vi "PH_ImageOperator.evt call set Fillfactor Settings.vi"(0 "i ref in":refnum<vi>, 1 "Instance":string, 2 "Calculate":bool, 3 "Threshold":dbl, 4 "Damage Threshold [J/cm²]":dbl, 5 "error in (no error)":errorcluster, 7 "Filter?":bool) -> (14 "i ref out":refnum<vi>, 19 "error out":errorcluster)   [LabVIEW 2014, in "PH_ImageOperator.lvlib"]
doc: "This VI calls the event case \"SetFFSettings\" by a simple call."
uses:
  PH_ImageOperator.lvlib
  CS_Core/CSSystem/CoreLib/CoreLib.double 2 byte array.vi
  CS_Core/CSSystem/CoreLib/CoreLib.short 2 byte array.vi
  CS_Core/CSSystem/CoreLib/CoreLib.lvlib
  CS_Core/BaseProcess/BaseProcess.lvlib
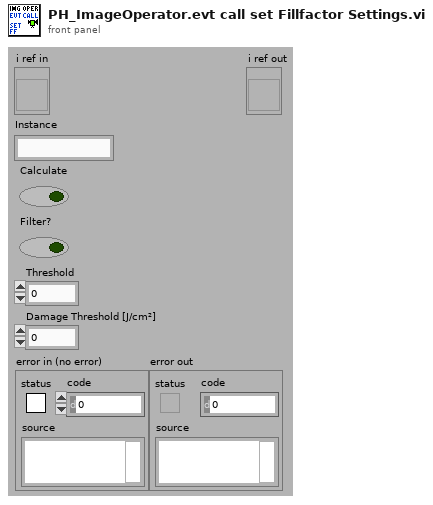
[diagram p1: front panel]
types:
  T1 = typedef "CoreDefs.rawDataType.ctl" = i8[]
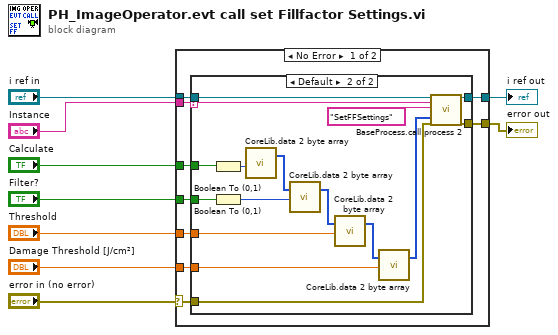
[diagram p0: block diagram]
diagram:
  n1 = case shown="No Error" "error in (no error)" {
    selector: "error in (no error)" -> [w14 w37]
    tunnel: [w18 w38] -> w8
    tunnel: [w17 w37] -> w7
    tunnel: "i ref in" -> [w16 w38]
    tunnel: "Instance" -> [w13 _]
    tunnel: "Calculate" -> [w15 _]
    tunnel: "Threshold" -> [w12 _]
    tunnel: "Damage Threshold [J/cm²]" -> [w11 _]
    tunnel: "Filter?" -> [w10 _]
    frame No Error {
      n2 = case shown="Default" w13 {
        selector: w13 -> [_ w21]
        tunnel: [w20 w35] -> w18
        tunnel: [w19 w34] -> w17
        tunnel: w16 -> [w20 w33]
        tunnel: w15 -> [_ w31]
        tunnel: w14 -> [w19 w30]
        tunnel: w12 -> [_ w27]
        tunnel: w11 -> [_ w26]
        tunnel: w10 -> [_ w23]
        frame "N/A" {
        }
        frame Default {
          n3 = Boolean To (0,1)(Boolean=w31) -> (0, 1=w32:i16)
          n4 = Boolean To (0,1)(Boolean=w23) -> (0, 1=w22:i16)
          n5 = call-poly "CoreLib.data 2 byte array.vi"("i16"=w32) -> ("byteArray out"=w25:T1)  [unwired: 18 in]
          n6 = call-poly "CoreLib.data 2 byte array.vi"("byteArray"=w25, "i16"=w22) -> ("byteArray out"=w24:T1)  [unwired: 17 in]
          n7 = call-poly "CoreLib.data 2 byte array.vi"("byteArray"=w24, "f64"=w27) -> ("byteArray out"=w29:T1)  [unwired: 17 in]
          n8 = call-poly "CoreLib.data 2 byte array.vi"("byteArray"=w29, "f64"=w26) -> ("byteArray out"=w28:T1)  [unwired: 17 in]
          n9 = call "BaseProcess.call process 2.vi"("i ref in"=w33, "Object"=w21, "Selector"="SetFFSettings", "Data"=w28, "error in (no error)"=w30) -> ("i ref out"=w35:refnum<vi>, "error out"=w34:errorcluster)  [unwired: 13 in]
        }
      }
    }
    frame Error {
    }
  }
  "i ref out" <- w8
  "error out" <- w7
